vi "Lab Panel V5.23.vi"() -> ()   [LabVIEW 2013] (continued)
                    n2497 = local read "DISP LAB05-2"() -> (w4651:T4)
                    n2498 = local read "SIG LAB05-2"() -> (w4652:T2)
                    n2499 = local read "ON L05-2"() -> (w4648:cluster{"amps":dbl, "volts":dbl, "pf":dbl})
                    n2500 = Unbundle(w4652) -> ("AMPS"=w4658:dbl, "VOLTS"=w4656:dbl, "PF"=w4655:dbl, "Tmp Live"=w4654:dbl, "Tmp Neut"=w4657:dbl)
                    n2501 = Unbundle(w4651) -> ("CYCLE"=w4653:dbl)  [unwired: 2 out]
                    n2502 = stacked-sequence {
                      tunnel: w4658 -> [w4662 w4681]
                      tunnel: w4657 -> [_ w4680]
                      tunnel: w4656 -> [w4661 w4679]
                      tunnel: w4655 -> [w4660 w4678]
                      tunnel: w4654 -> [_ w4677]
                      tunnel: w4653 -> [_ w4676]
                      tunnel: w4650 -> [_ w4675]
                      tunnel: w4649 -> [w4663 _]
                      tunnel: w4648 -> [w4659 w4673]
                      tunnel: w4647 -> [_ w4674]
                      tunnel: w4646 -> [_ w4669]
                      frame #0 {
                        n2503 = case shown="True" w4663 {
                          tunnel: w4662 -> [_ w4668]
                          tunnel: w4661 -> [_ w4667]
                          tunnel: w4660 -> [_ w4666]
                          tunnel: w4659 -> [_ w4664]
                          frame False {
                          }
                          frame True {
                            n2504 = Bundle(cluster=w4664, "amps"=w4668, "volts"=w4667, "pf"=w4666) -> (w4665:cluster{"amps":dbl, "volts":dbl, "pf":dbl})
                            n2505 = local write "ON L05-2"(w4665) -> ()
                          }
                        }
                      }
                      frame #1 {
                        n2506 = Unbundle(w4673) -> ("amps"=w4672:dbl, "volts"=w4671:dbl, "pf"=w4670:dbl)
                        n2507 = case shown="True" w4674 {
                          tunnel: w4681 -> [_ w4713]
                          tunnel: w4680 -> [_ w4720]
                          tunnel: w4679 -> [_ _]
                          tunnel: w4678 -> [_ _]
                          tunnel: w4677 -> [_ w4719]
                          tunnel: w4676 -> [_ w4718]
                          tunnel: w4675 -> [_ w4683]
                          tunnel: w4672 -> [_ w4715]
                          tunnel: w4671 -> [_ w4714]
                          tunnel: w4670 -> [_ w4712]
                          tunnel: w4669 -> [_ w4704]
                          frame False {
                          }
                          frame True {
                            n2508 = local read "TDMS LAB05-2"() -> (w4717:refnum<k34>)
                            n2509 = Build Array(w4714) -> (w4709:dbl[])
                            n2510 = Build Array(w4712) -> (w4708:dbl[])
                            n2511 = Build Array(w4719) -> (w4707:dbl[])
                            n2512 = Build Array(w4720) -> (w4706:dbl[])
                            n2513 = Build Array(w4715) -> (w4711:dbl[])
                            n2514 = Build Array(w4713) -> (w4710:dbl[])
                            n2515 = Build Array(w4718) -> (w4705:dbl[])
                            n2516 = Build Array("AMPS ON", "AMPS OFF", "VOLTS", "PF", "TEMP Live", "TEMP Neut", "CYCLE") -> (w4688:string[])
                            n2517 = Bundle By Name("Y"=w4711, "t0"=w4704) -> (w4703:waveform(dbl))  [unwired: 1 in]
                            n2518 = Bundle By Name("Y"=w4710, "t0"=w4704) -> (w4702:waveform(dbl))  [unwired: 1 in]
                            n2519 = Bundle By Name("Y"=w4709, "t0"=w4704) -> (w4701:waveform(dbl))  [unwired: 1 in]
                            n2520 = Bundle By Name("Y"=w4708, "t0"=w4704) -> (w4700:waveform(dbl))  [unwired: 1 in]
                            n2521 = Bundle By Name("Y"=w4707, "t0"=w4704) -> (w4699:waveform(dbl))  [unwired: 1 in]
                            n2522 = Bundle By Name("Y"=w4706, "t0"=w4704) -> (w4698:waveform(dbl))  [unwired: 1 in]
                            n2523 = Bundle By Name("Y"=w4705, "t0"=w4704) -> (w4697:waveform(dbl))  [unwired: 1 in]
                            n2524 = Build Array(w4703, w4702, w4701, w4700, w4699, w4698, w4697) -> (w4696:waveform(dbl)[])
                            n2525 = TDMS Write(0:w4717, 5:"TEST VALUES", 7:w4688, 9:w4696) -> (4:w4687:refnum<k34>, 6:w4686:string, 15:w4685:errorcluster)  [unwired: 2 in, 1 out]
                            n2526 = TDMS Write(0:w4687, 5:w4686, 7:"TIME", 9:w4683, 11:w4685) -> (15:w4682:errorcluster)  [unwired: 1 in, 3 out]
                            n2527 = local write "data file error"(w4682) -> ()
                          }
                        }
                      }
                    }
                  }
                }
              }
            }
          }
          frame #13 {
            # "display test values on chart"
            n2528 = local read "jig cycle"() -> (w4725:dbl)
            n2529 = local read "on loops"() -> (w4727:dbl)
            n2530 = Add(x=w4727, y=2) -> (x+y=w4724:dbl)
            n2531 = Equal?(x=w4725, y=1) -> (x = y?=w4723:bool)
            n2532 = Equal?(x=w4725, y=w4724) -> (x = y?=w4722:bool)
            n2533 = Or(x=w4723, y=w4722) -> (x .or. y?=w4721:bool)
            "graph flag" <- w4721
            n2534 = global write "Global display 3.vi" "graph flag"(w4721) -> ()
            n2535 = case shown="True" w4721 {
              frame False {
              }
              frame True {
                n2536 = local read "SIG LAB05-1"() -> (w4770:T2)
                n2537 = local read "SIG LAB04-2"() -> (w4771:T2)
                n2538 = local read "SIG LAB05-2"() -> (w4769:T2)
                n2539 = local read "SIG LAB04-1"() -> (w4772:T2)
                n2540 = local read "SIG LAB03-1"() -> (w4774:T2)
                n2541 = local read "SIG LAB03-2"() -> (w4773:T2)
                n2542 = local read "SIG LAB01-1"() -> (w4778:T2)
                n2543 = local read "SIG LAB02-2"() -> (w4775:T2)
                n2544 = local read "SIG LAB02-1"() -> (w4776:T2)
                n2545 = local read "SIG LAB01-2"() -> (w4777:T2)
                n2546 = Unbundle(w4771) -> ("AMPS"=w4761:dbl, "VOLTS"=w4751:dbl, "Tmp Live"=w4741:dbl, "Tmp Neut"=w4731:dbl)  [unwired: 1 out]
                n2547 = Unbundle(w4770) -> ("AMPS"=w4760:dbl, "VOLTS"=w4750:dbl, "Tmp Live"=w4740:dbl, "Tmp Neut"=w4730:dbl)  [unwired: 1 out]
                n2548 = Unbundle(w4769) -> ("AMPS"=w4759:dbl, "VOLTS"=w4749:dbl, "Tmp Live"=w4739:dbl, "Tmp Neut"=w4729:dbl)  [unwired: 1 out]
                n2549 = Unbundle(w4772) -> ("AMPS"=w4762:dbl, "VOLTS"=w4752:dbl, "Tmp Live"=w4742:dbl, "Tmp Neut"=w4732:dbl)  [unwired: 1 out]
                n2550 = Unbundle(w4773) -> ("AMPS"=w4763:dbl, "VOLTS"=w4753:dbl, "Tmp Live"=w4743:dbl, "Tmp Neut"=w4733:dbl)  [unwired: 1 out]
                n2551 = Unbundle(w4774) -> ("AMPS"=w4764:dbl, "VOLTS"=w4754:dbl, "Tmp Live"=w4744:dbl, "Tmp Neut"=w4734:dbl)  [unwired: 1 out]
                n2552 = Unbundle(w4775) -> ("AMPS"=w4765:dbl, "VOLTS"=w4755:dbl, "Tmp Live"=w4745:dbl, "Tmp Neut"=w4735:dbl)  [unwired: 1 out]
                n2553 = Unbundle(w4776) -> ("AMPS"=w4766:dbl, "VOLTS"=w4756:dbl, "Tmp Live"=w4746:dbl, "Tmp Neut"=w4736:dbl)  [unwired: 1 out]
                n2554 = Unbundle(w4778) -> ("AMPS"=w4768:dbl, "VOLTS"=w4758:dbl, "Tmp Live"=w4748:dbl, "Tmp Neut"=w4738:dbl)  [unwired: 1 out]
                n2555 = Unbundle(w4777) -> ("AMPS"=w4767:dbl, "VOLTS"=w4757:dbl, "Tmp Live"=w4747:dbl, "Tmp Neut"=w4737:dbl)  [unwired: 1 out]
                n2556 = stacked-sequence {
                  tunnel: w4768 -> [w4810 _ _]
                  tunnel: w4767 -> [w4809 _ _]
                  tunnel: w4766 -> [w4800 _ _]
                  tunnel: w4765 -> [w4799 _ _]
                  tunnel: w4764 -> [w4789 _ _]
                  tunnel: w4763 -> [w4788 _ _]
                  tunnel: w4762 -> [_ w4833 _]
                  tunnel: w4761 -> [_ w4832 _]
                  tunnel: w4760 -> [_ w4822 _]
                  tunnel: w4759 -> [_ w4821 _]
                  tunnel: w4758 -> [w4807 _ _]
                  tunnel: w4757 -> [w4806 _ _]
                  tunnel: w4756 -> [w4797 _ _]
                  tunnel: w4755 -> [w4796 _ _]
                  tunnel: w4754 -> [w4787 _ _]
                  tunnel: w4753 -> [w4786 _ _]
                  tunnel: w4752 -> [_ w4831 _]
                  tunnel: w4751 -> [_ w4830 _]
                  tunnel: w4750 -> [_ w4820 _]
                  tunnel: w4749 -> [_ w4819 _]
                  tunnel: w4748 -> [w4804 _ _]
                  tunnel: w4747 -> [w4802 _ _]
                  tunnel: w4746 -> [w4793 _ _]
                  tunnel: w4745 -> [w4791 _ _]
                  tunnel: w4744 -> [w4785 _ _]
                  tunnel: w4743 -> [w4783 _ _]
                  tunnel: w4742 -> [_ w4829 _]
                  tunnel: w4741 -> [_ w4827 _]
                  tunnel: w4740 -> [_ w4818 _]
                  tunnel: w4739 -> [_ w4816 _]
                  tunnel: w4738 -> [w4803 _ _]
                  tunnel: w4737 -> [w4801 _ _]
                  tunnel: w4736 -> [w4792 _ _]
                  tunnel: w4735 -> [w4790 _ _]
                  tunnel: w4734 -> [w4784 _ _]
                  tunnel: w4733 -> [w4782 _ _]
                  tunnel: w4732 -> [_ w4828 _]
                  tunnel: w4731 -> [_ w4826 _]
                  tunnel: w4730 -> [_ w4817 _]
                  tunnel: w4729 -> [_ w4815 _]
                  frame #0 {
                    n2557 = Merge Signals(w4810, w4809) -> (→"LAB01 AMPS":dynamicdata)
                    n2558 = Merge Signals(w4807, w4806) -> (→"LAB01 VOLTS":dynamicdata)
                    n2559 = Merge Signals(w4787, w4786) -> (→"LAB03 VOLTS":dynamicdata)
                    n2560 = Merge Signals(w4804, w4803, w4802, w4801) -> (→"LAB01 deg C":dynamicdata)
                    n2561 = Merge Signals(w4800, w4799) -> (→"LAB02 AMPS":dynamicdata)
                    n2562 = Merge Signals(w4793, w4792, w4791, w4790) -> (→"LAB02 deg C":dynamicdata)
                    n2563 = Merge Signals(w4785, w4784, w4783, w4782) -> (→"LAB03 deg C":dynamicdata)
                    n2564 = Merge Signals(w4797, w4796) -> (→"LAB02 VOLTS":dynamicdata)
                    n2565 = Merge Signals(w4789, w4788) -> (→"LAB03 AMPS":dynamicdata)
                  }
                  frame #1 {
                    n2566 = Merge Signals(w4820, w4819) -> (→"LAB05 VOLTS":dynamicdata)
                    n2567 = Merge Signals(w4833, w4832) -> (→"LAB04 AMPS":dynamicdata)
                    n2568 = Merge Signals(w4822, w4821) -> (→"LAB05 AMPS":dynamicdata)
                    n2569 = Merge Signals(w4818, w4817, w4816, w4815) -> (→"LAB05 deg C":dynamicdata)
                    n2570 = Merge Signals(w4829, w4828, w4827, w4826) -> (→"LAB04 deg C":dynamicdata)
                    n2571 = Merge Signals(w4831, w4830) -> (→"LAB04 VOLTS":dynamicdata)
                  }
                  frame #2 {
                    n2572 = local read "LAB05 VOLTS"() -> (w4841:dynamicdata)
                    n2573 = local read "LAB04 VOLTS"() -> (w4842:dynamicdata)
                    n2574 = local read "LAB02 VOLTS"() -> (w4844:dynamicdata)
                    n2575 = local read "LAB03 VOLTS"() -> (w4843:dynamicdata)
                    n2576 = local read "LAB05 AMPS"() -> (w4847:dynamicdata)
                    n2577 = local read "LAB01 VOLTS"() -> (w4845:dynamicdata)
                    n2578 = local read "LAB04 AMPS"() -> (w4848:dynamicdata)
                    n2579 = local read "LAB03 AMPS"() -> (w4849:dynamicdata)
                    n2580 = local read "LAB03 deg C"() -> (w4837:dynamicdata)
                    n2581 = local read "LAB02 AMPS"() -> (w4850:dynamicdata)
                    n2582 = local read "LAB04 deg C"() -> (w4836:dynamicdata)
                    n2583 = local read "LAB05 deg C"() -> (w4835:dynamicdata)
                    n2584 = local read "LAB02 deg C"() -> (w4838:dynamicdata)
                    n2585 = local read "LAB01 deg C"() -> (w4839:dynamicdata)
                    n2586 = local read "LAB01 AMPS"() -> (w4851:dynamicdata)
                    n2587 = Merge Signals(w4839, w4838, w4837, w4836, w4835) -> (w4834:dynamicdata)
                    n2588 = Merge Signals(w4851, w4850, w4849, w4848, w4847) -> (w4846:dynamicdata)
                    n2589 = Merge Signals(w4845, w4844, w4843, w4842, w4841) -> (w4840:dynamicdata)
                    n2590 = global write "Global display 3.vi" "graph volts"(w4840) -> ()
                    n2591 = global write "Global display 3.vi" "graph deg C"(w4834) -> ()
                    n2592 = global write "Global display 3.vi" "graph amps"(w4846) -> ()
                  }
                }
              }
            }
          }
          frame #14 {
            # "check for amps fail"
            # "check for cycle test & temperature rise fail conditions"
            n2593 = local read "on loops"() -> (w4878:dbl)
            n2594 = local read "jig cycle"() -> (w4875:dbl)
            n2595 = local read "jig cycle"() -> (w4880:dbl)
            n2596 = Add(x=w4878, y=3.0) -> (x+y=w4876:dbl)
            n2597 = Equal?(x=w4875, y=w4876) -> (x = y?=w4871:bool)
            n2598 = local read "Fail Loops"() -> (w4852:dbl)
            n2599 = Equal?(x=w4880, y=1.0) -> (x = y?=w4873:bool)
            n2600 = global write "Global 1.vi" "fail count"(w4852) -> ()
            n2601 = stacked-sequence {
              tunnel: w4874 -> [w4883 _ _ _ _ _ _ _ _ _]
              tunnel: w4873 -> [w4884 w4904 w4924 w4944 w4964 w4984 w5004 w5024 w5044 w5064]
              tunnel: w4872 -> [w4881 _ _ _ _ _ _ _ _ _]
              tunnel: w4871 -> [w4882 w4903 w4923 w4943 w4963 w4983 w5003 w5023 w5043 w5063]
              tunnel: w4870 -> [_ w4902 _ _ _ _ _ _ _ _]
              tunnel: w4869 -> [_ w4901 _ _ _ _ _ _ _ _]
              tunnel: w4868 -> [_ _ w4922 _ _ _ _ _ _ _]
              tunnel: w4867 -> [_ _ w4921 _ _ _ _ _ _ _]
              tunnel: w4866 -> [_ _ _ w4942 _ _ _ _ _ _]
              tunnel: w4865 -> [_ _ _ w4941 _ _ _ _ _ _]
              tunnel: w4864 -> [_ _ _ _ w4962 _ _ _ _ _]
              tunnel: w4863 -> [_ _ _ _ w4961 _ _ _ _ _]
              tunnel: w4862 -> [_ _ _ _ _ w4982 _ _ _ _]
              tunnel: w4861 -> [_ _ _ _ _ w4981 _ _ _ _]
              tunnel: w4860 -> [_ _ _ _ _ _ w5002 _ _ _]
              tunnel: w4859 -> [_ _ _ _ _ _ w5001 _ _ _]
              tunnel: w4858 -> [_ _ _ _ _ _ _ w5022 _ _]
              tunnel: w4857 -> [_ _ _ _ _ _ _ w5021 _ _]
              tunnel: w4856 -> [_ _ _ _ _ _ _ _ w5042 _]
              tunnel: w4855 -> [_ _ _ _ _ _ _ _ w5041 _]
              tunnel: w4854 -> [_ _ _ _ _ _ _ _ _ w5062]
              tunnel: w4853 -> [_ _ _ _ _ _ _ _ _ w5061]
              frame #0 {
                # "LAB01-1"
                n2602 = case shown="True" w4881 {
                  tunnel: w4884 -> [_ w4897]
                  tunnel: w4883 -> [_ w4894]
                  tunnel: w4882 -> [_ w4893]
                  frame False {
                  }
                  frame True {
                    n2603 = local read "TEMP START LAB01-1"() -> (w4899:cluster{"TL":dbl, "TN":dbl})
                    n2604 = local read "RESULT LAB01-1"() -> (w4888:bool)
                    n2605 = local read "FAIL LAB01-1"() -> (w4891:cluster{"LO":dbl, "HI":dbl})
                    n2606 = local read "TDMS LAB01-1"() -> (w4898:refnum<k34>)
                    n2607 = local read "SET LAB01-1"() -> (w4895:T5)
                    n2608 = local read "DISP LAB01-1"() -> (w4896:T4)
                    n2609 = local read "SIG LAB01-1"() -> (w4900:T2)
                    n2610 = Bundle("FAIL LAB01-1"=w4891, "SIG LAB01-1"=w4900, "TEMP START LAB01-1"=w4899, "DISP LAB01-1"=w4896, "SET LAB01-1"=w4895, "TDMS LAB01-1"=w4898) -> (w4885:T33)  [unwired: 1 in]
                    n2611 = call "sub vi - cycle&temp fail v7.vi"("Amps Lo?"=w4897, "Input Cluster"=w4885, "SELECT"=w4894, "Amps Hi?"=w4893, "Result In"=w4888) -> ("(FAIL) out"=w4890:cluster{"FAIL LO":dbl, "FAIL HI":dbl}, "(DISP) out"=w4886:T4, "T-RISE"=w4887:cluster{"T-RISE (L)":dbl, "T-RISE (N)":dbl}, "Result Out"=w4889:bool, "file error"=w4892:errorcluster)  [unwired: 10 in]
                    n2612 = local write "TEMP RISE LAB01-1"(w4887) -> ()
                    n2613 = local write "FAIL LAB01-1"(w4890) -> ()
                    n2614 = local write "DISP LAB01-1"(w4886) -> ()
                    n2615 = local write "RESULT LAB01-1"(w4889) -> ()
                    n2616 = local write "data file error"(w4892) -> ()
                  }
                }
              }
              frame #1 {
                # "LAB01-2"
                n2617 = case shown="True" w4902 {
                  tunnel: w4904 -> [_ w4917]
                  tunnel: w4901 -> [_ w4914]
                  tunnel: w4903 -> [_ w4913]
                  frame False {
                  }
                  frame True {
                    n2618 = local read "TEMP START LAB01-2"() -> (w4919:cluster{"TL":dbl, "TN":dbl})
                    n2619 = local read "FAIL LAB01-2"() -> (w4910:cluster{"LO":dbl, "HI":dbl})
                    n2620 = local read "TDMS LAB01-2"() -> (w4918:refnum<k34>)
                    n2621 = local read "SET LAB01-2"() -> (w4915:T5)
                    n2622 = local read "DISP LAB01-2"() -> (w4916:T4)
                    n2623 = local read "RESULT LAB01-2"() -> (w4907:bool)
                    n2624 = local read "SIG LAB01-2"() -> (w4920:T2)
                    n2625 = Bundle("FAIL LAB01-2"=w4910, "SIG LAB01-2"=w4920, "TEMP START LAB01-2"=w4919, "DISP LAB01-2"=w4916, "SET LAB01-2"=w4915, "TDMS LAB01-2"=w4918) -> (w4905:T34)  [unwired: 1 in]
                    n2626 = call "sub vi - cycle&temp fail v7.vi"("Amps Lo?"=w4917, "Input Cluster"=w4905, "SELECT"=w4914, "Amps Hi?"=w4913, "Result In"=w4907) -> ("(FAIL) out"=w4909:cluster{"FAIL LO":dbl, "FAIL HI":dbl}, "(DISP) out"=w4912:T4, "T-RISE"=w4906:cluster{"T-RISE (L)":dbl, "T-RISE (N)":dbl}, "Result Out"=w4908:bool, "file error"=w4911:errorcluster)  [unwired: 10 in]
                    n2627 = local write "TEMP RISE LAB01-2"(w4906) -> ()
                    n2628 = local write "FAIL LAB01-2"(w4909) -> ()
                    n2629 = local write "DISP LAB01-2"(w4912) -> ()
                    n2630 = local write "RESULT LAB01-2"(w4908) -> ()
                    n2631 = local write "data file error"(w4911) -> ()
                  }
                }
              }
              frame #2 {
                # "LAB02-1"
                n2632 = case shown="True" w4922 {
                  tunnel: w4924 -> [_ w4937]
                  tunnel: w4921 -> [_ w4934]
                  tunnel: w4923 -> [_ w4933]
                  frame False {
                  }
                  frame True {
                    n2633 = local read "TEMP START LAB02-1"() -> (w4939:cluster{"TL":dbl, "TN":dbl})
                    n2634 = local read "FAIL LAB02-1"() -> (w4930:cluster{"LO":dbl, "HI":dbl})
                    n2635 = local read "TDMS LAB02-1"() -> (w4938:refnum<k34>)
                    n2636 = local read "SET LAB02-1"() -> (w4935:T5)
                    n2637 = local read "DISP LAB02-1"() -> (w4936:T4)
                    n2638 = local read "SIG LAB02-1"() -> (w4940:T2)
                    n2639 = local read "RESULT LAB02-1"() -> (w4927:bool)
                    n2640 = Bundle("FAIL LAB02-1"=w4930, "SIG LAB02-1"=w4940, "TEMP START LAB02-1"=w4939, "DISP LAB02-1"=w4936, "SET LAB02-1"=w4935, "TDMS LAB02-1"=w4938) -> (w4925:T35)  [unwired: 1 in]
                    n2641 = call "sub vi - cycle&temp fail v7.vi"("Amps Lo?"=w4937, "Input Cluster"=w4925, "SELECT"=w4934, "Amps Hi?"=w4933, "Result In"=w4927) -> ("(FAIL) out"=w4929:cluster{"FAIL LO":dbl, "FAIL HI":dbl}, "(DISP) out"=w4932:T4, "T-RISE"=w4926:cluster{"T-RISE (L)":dbl, "T-RISE (N)":dbl}, "Result Out"=w4928:bool, "file error"=w4931:errorcluster)  [unwired: 10 in]
                    n2642 = local write "TEMP RISE LAB02-1"(w4926) -> ()
                    n2643 = local write "FAIL LAB02-1"(w4929) -> ()
                    n2644 = local write "DISP LAB02-1"(w4932) -> ()
                    n2645 = local write "RESULT LAB02-1"(w4928) -> ()
                    n2646 = local write "data file error"(w4931) -> ()
                  }
                }
              }
              frame #3 {
                # "LAB02-2"
                n2647 = case shown="True" w4942 {
                  tunnel: w4944 -> [_ w4957]
                  tunnel: w4941 -> [_ w4954]
                  tunnel: w4943 -> [_ w4953]
                  frame False {
                  }
                  frame True {
                    n2648 = local read "TEMP START LAB02-2"() -> (w4959:cluster{"TL":dbl, "TN":dbl})
                    n2649 = local read "FAIL LAB02-2"() -> (w4950:cluster{"LO":dbl, "HI":dbl})
                    n2650 = local read "TDMS LAB02-2"() -> (w4958:refnum<k34>)
                    n2651 = local read "SET LAB02-2"() -> (w4955:T5)
                    n2652 = local read "DISP LAB02-2"() -> (w4956:T4)
                    n2653 = local read "SIG LAB02-2"() -> (w4960:T2)
                    n2654 = local read "RESULT LAB02-2"() -> (w4947:bool)
                    n2655 = Bundle("FAIL LAB02-2"=w4950, "SIG LAB02-2"=w4960, "TEMP START LAB02-2"=w4959, "DISP LAB02-2"=w4956, "SET LAB02-2"=w4955, "TDMS LAB02-2"=w4958) -> (w4945:T36)  [unwired: 1 in]
                    n2656 = call "sub vi - cycle&temp fail v7.vi"("Amps Lo?"=w4957, "Input Cluster"=w4945, "SELECT"=w4954, "Amps Hi?"=w4953, "Result In"=w4947) -> ("(FAIL) out"=w4949:cluster{"FAIL LO":dbl, "FAIL HI":dbl}, "(DISP) out"=w4952:T4, "T-RISE"=w4946:cluster{"T-RISE (L)":dbl, "T-RISE (N)":dbl}, "Result Out"=w4948:bool, "file error"=w4951:errorcluster)  [unwired: 10 in]
                    n2657 = local write "TEMP RISE LAB02-2"(w4946) -> ()
                    n2658 = local write "FAIL LAB02-2"(w4949) -> ()
                    n2659 = local write "DISP LAB02-2"(w4952) -> ()
                    n2660 = local write "RESULT LAB02-2"(w4948) -> ()
                    n2661 = local write "data file error"(w4951) -> ()
                  }
                }
              }
              frame #4 {
                # "LAB03-1"
                n2662 = case shown="True" w4962 {
                  tunnel: w4964 -> [_ w4977]
                  tunnel: w4961 -> [_ w4974]
                  tunnel: w4963 -> [_ w4973]
                  frame False {
                  }
                  frame True {
                    n2663 = local read "TEMP START LAB03-1"() -> (w4979:cluster{"TL":dbl, "TN":dbl})
                    n2664 = local read "FAIL LAB03-1"() -> (w4970:cluster{"LO":dbl, "HI":dbl})
                    n2665 = local read "TDMS LAB03-1"() -> (w4978:refnum<k34>)
                    n2666 = local read "SET LAB03-1"() -> (w4975:T5)
                    n2667 = local read "DISP LAB03-1"() -> (w4976:T4)
                    n2668 = local read "SIG LAB03-1"() -> (w4980:T2)
                    n2669 = local read "RESULT LAB03-1"() -> (w4967:bool)
                    n2670 = Bundle("FAIL LAB03-1"=w4970, "SIG LAB03-1"=w4980, "TEMP START LAB03-1"=w4979, "DISP LAB03-1"=w4976, "SET LAB03-1"=w4975, "TDMS LAB03-1"=w4978) -> (w4965:T37)  [unwired: 1 in]
                    n2671 = call "sub vi - cycle&temp fail v7.vi"("Amps Lo?"=w4977, "Input Cluster"=w4965, "SELECT"=w4974, "Amps Hi?"=w4973, "Result In"=w4967) -> ("(FAIL) out"=w4969:cluster{"FAIL LO":dbl, "FAIL HI":dbl}, "(DISP) out"=w4972:T4, "T-RISE"=w4966:cluster{"T-RISE (L)":dbl, "T-RISE (N)":dbl}, "Result Out"=w4968:bool, "file error"=w4971:errorcluster)  [unwired: 10 in]
                    n2672 = local write "TEMP RISE LAB03-1"(w4966) -> ()
                    n2673 = local write "FAIL LAB03-1"(w4969) -> ()
                    n2674 = local write "DISP LAB03-1"(w4972) -> ()
                    n2675 = local write "RESULT LAB03-1"(w4968) -> ()
                    n2676 = local write "data file error"(w4971) -> ()
                  }
                }
              }
              frame #5 {
                # "LAB03-2"
                n2677 = case shown="True" w4982 {
                  tunnel: w4984 -> [_ w4997]
                  tunnel: w4981 -> [_ w4994]
                  tunnel: w4983 -> [_ w4993]
                  frame False {
                  }
                  frame True {
                    n2678 = local read "TEMP START LAB03-2"() -> (w4999:cluster{"TL":dbl, "TN":dbl})
                    n2679 = local read "FAIL LAB03-2"() -> (w4990:cluster{"LO":dbl, "HI":dbl})
                    n2680 = local read "TDMS LAB03-2"() -> (w4998:refnum<k34>)
                    n2681 = local read "SET LAB03-2"() -> (w4995:T5)
                    n2682 = local read "DISP LAB03-2"() -> (w4996:T4)
                    n2683 = local read "RESULT LAB03-2"() -> (w4987:bool)
                    n2684 = local read "SIG LAB03-2"() -> (w5000:T2)
                    n2685 = Bundle("FAIL LAB03-2"=w4990, "SIG LAB03-2"=w5000, "TEMP START LAB03-2"=w4999, "DISP LAB03-2"=w4996, "SET LAB03-2"=w4995, "TDMS LAB03-2"=w4998) -> (w4985:T38)  [unwired: 1 in]
                    n2686 = call "sub vi - cycle&temp fail v7.vi"("Amps Lo?"=w4997, "Input Cluster"=w4985, "SELECT"=w4994, "Amps Hi?"=w4993, "Result In"=w4987) -> ("(FAIL) out"=w4989:cluster{"FAIL LO":dbl, "FAIL HI":dbl}, "(DISP) out"=w4992:T4, "T-RISE"=w4986:cluster{"T-RISE (L)":dbl, "T-RISE (N)":dbl}, "Result Out"=w4988:bool, "file error"=w4991:errorcluster)  [unwired: 10 in]
                    n2687 = local write "FAIL LAB03-2"(w4989) -> ()
                    n2688 = local write "TEMP RISE LAB03-2"(w4986) -> ()
                    n2689 = local write "DISP LAB03-2"(w4992) -> ()
                    n2690 = local write "RESULT LAB03-2"(w4988) -> ()
                    n2691 = local write "data file error"(w4991) -> ()
                  }
                }
              }
              frame #6 {
                # "LAB04-1"
                n2692 = case shown="True" w5002 {
                  tunnel: w5004 -> [_ w5017]
                  tunnel: w5001 -> [_ w5014]
                  tunnel: w5003 -> [_ w5013]
                  frame False {
                  }
                  frame True {
                    n2693 = local read "TEMP START LAB04-1"() -> (w5019:cluster{"TL":dbl, "TN":dbl})
                    n2694 = local read "FAIL LAB04-1"() -> (w5010:cluster{"LO":dbl, "HI":dbl})
                    n2695 = local read "TDMS LAB04-1"() -> (w5018:refnum<k34>)
                    n2696 = local read "SET LAB04-1"() -> (w5015:T5)
                    n2697 = local read "DISP LAB04-1"() -> (w5016:T4)
                    n2698 = local read "SIG LAB04-1"() -> (w5020:T2)
                    n2699 = local read "RESULT LAB04-1"() -> (w5007:bool)
                    n2700 = Bundle("FAIL LAB04-1"=w5010, "SIG LAB04-1"=w5020, "TEMP START LAB04-1"=w5019, "DISP LAB04-1"=w5016, "SET LAB04-1"=w5015, "TDMS LAB04-1"=w5018) -> (w5005:T39)  [unwired: 1 in]
                    n2701 = call "sub vi - cycle&temp fail v7.vi"("Amps Lo?"=w5017, "Input Cluster"=w5005, "SELECT"=w5014, "Amps Hi?"=w5013, "Result In"=w5007) -> ("(FAIL) out"=w5009:cluster{"FAIL LO":dbl, "FAIL HI":dbl}, "(DISP) out"=w5012:T4, "T-RISE"=w5006:cluster{"T-RISE (L)":dbl, "T-RISE (N)":dbl}, "Result Out"=w5008:bool, "file error"=w5011:errorcluster)  [unwired: 10 in]
                    n2702 = local write "TEMP RISE LAB04-1"(w5006) -> ()
                    n2703 = local write "FAIL LAB04-1"(w5009) -> ()
                    n2704 = local write "DISP LAB04-1"(w5012) -> ()
                    n2705 = local write "RESULT LAB04-1"(w5008) -> ()
                    n2706 = local write "data file error"(w5011) -> ()
                  }
                }
              }
              frame #7 {
                # "LAB04-2"
                n2707 = case shown="True" w5022 {
                  tunnel: w5024 -> [_ w5037]
                  tunnel: w5021 -> [_ w5034]
                  tunnel: w5023 -> [_ w5033]
                  frame False {
                  }
                  frame True {
                    n2708 = local read "TEMP START LAB04-2"() -> (w5039:cluster{"TL":dbl, "TN":dbl})
                    n2709 = local read "FAIL LAB04-2"() -> (w5030:cluster{"LO":dbl, "HI":dbl})
                    n2710 = local read "TDMS LAB04-2"() -> (w5038:refnum<k34>)
                    n2711 = local read "SET LAB04-2"() -> (w5035:T5)
                    n2712 = local read "DISP LAB04-2"() -> (w5036:T4)
                    n2713 = local read "SIG LAB04-2"() -> (w5040:T2)
                    n2714 = local read "RESULT LAB04-2"() -> (w5027:bool)
                    n2715 = Bundle("FAIL LAB04-2"=w5030, "SIG LAB04-2"=w5040, "TEMP START LAB04-2"=w5039, "DISP LAB04-2"=w5036, "SET LAB04-2"=w5035, "TDMS LAB04-2"=w5038) -> (w5025:T40)  [unwired: 1 in]
                    n2716 = call "sub vi - cycle&temp fail v7.vi"("Amps Lo?"=w5037, "Input Cluster"=w5025, "SELECT"=w5034, "Amps Hi?"=w5033, "Result In"=w5027) -> ("(FAIL) out"=w5029:cluster{"FAIL LO":dbl, "FAIL HI":dbl}, "(DISP) out"=w5032:T4, "T-RISE"=w5026:cluster{"T-RISE (L)":dbl, "T-RISE (N)":dbl}, "Result Out"=w5028:bool, "file error"=w5031:errorcluster)  [unwired: 10 in]
                    n2717 = local write "TEMP RISE LAB04-2"(w5026) -> ()
                    n2718 = local write "FAIL LAB04-2"(w5029) -> ()
                    n2719 = local write "DISP LAB04-2"(w5032) -> ()
                    n2720 = local write "RESULT LAB04-2"(w5028) -> ()
                    n2721 = local write "data file error"(w5031) -> ()
                  }
                }
              }
              frame #8 {
                # "LAB05-1"
                n2722 = case shown="True" w5042 {
                  tunnel: w5044 -> [_ w5057]
                  tunnel: w5041 -> [_ w5054]
                  tunnel: w5043 -> [_ w5053]
                  frame False {
                  }
                  frame True {
                    n2723 = local read "TEMP START LAB05-1"() -> (w5059:cluster{"TL":dbl, "TN":dbl})
                    n2724 = local read "FAIL LAB05-1"() -> (w5050:cluster{"LO":dbl, "HI":dbl})
                    n2725 = local read "TDMS LAB05-1"() -> (w5058:refnum<k34>)
                    n2726 = local read "SET LAB05-1"() -> (w5055:T5)
                    n2727 = local read "DISP LAB05-1"() -> (w5056:T4)
                    n2728 = local read "SIG LAB05-1"() -> (w5060:T2)
                    n2729 = local read "RESULT LAB05-1"() -> (w5047:bool)
                    n2730 = Bundle("FAIL LAB05-1"=w5050, "SIG LAB05-1"=w5060, "TEMP START LAB05-1"=w5059, "DISP LAB05-1"=w5056, "SET LAB05-1"=w5055, "TDMS LAB05-1"=w5058) -> (w5045:T41)  [unwired: 1 in]
                    n2731 = call "sub vi - cycle&temp fail v7.vi"("Amps Lo?"=w5057, "Input Cluster"=w5045, "SELECT"=w5054, "Amps Hi?"=w5053, "Result In"=w5047) -> ("(FAIL) out"=w5049:cluster{"FAIL LO":dbl, "FAIL HI":dbl}, "(DISP) out"=w5052:T4, "T-RISE"=w5046:cluster{"T-RISE (L)":dbl, "T-RISE (N)":dbl}, "Result Out"=w5048:bool, "file error"=w5051:errorcluster)  [unwired: 10 in]
                    n2732 = local write "TEMP RISE LAB05-1"(w5046) -> ()
                    n2733 = local write "FAIL LAB05-1"(w5049) -> ()
                    n2734 = local write "DISP LAB05-1"(w5052) -> ()
                    n2735 = local write "RESULT LAB05-1"(w5048) -> ()
                    n2736 = local write "data file error"(w5051) -> ()
                  }
                }
              }
              frame #9 {
                # "LAB05-2"
                n2737 = case shown="True" w5062 {
                  tunnel: w5064 -> [_ w5077]
                  tunnel: w5061 -> [_ w5074]
                  tunnel: w5063 -> [_ w5073]
                  frame False {
                  }
                  frame True {
                    n2738 = local read "TEMP START LAB05-2"() -> (w5079:cluster{"TL":dbl, "TN":dbl})
                    n2739 = local read "FAIL LAB05-2"() -> (w5070:cluster{"LO":dbl, "HI":dbl})
                    n2740 = local read "TDMS LAB05-2"() -> (w5078:refnum<k34>)
                    n2741 = local read "SET LAB05-2"() -> (w5075:T5)
                    n2742 = local read "DISP LAB05-2"() -> (w5076:T4)
                    n2743 = local read "SIG LAB05-2"() -> (w5080:T2)
                    n2744 = local read "RESULT LAB05-2"() -> (w5067:bool)
                    n2745 = Bundle("FAIL LAB05-2"=w5070, "SIG LAB05-2"=w5080, "TEMP START LAB05-2"=w5079, "DISP LAB05-2"=w5076, "SET LAB05-2"=w5075, "TDMS LAB05-2"=w5078) -> (w5065:T42)  [unwired: 1 in]
                    n2746 = call "sub vi - cycle&temp fail v7.vi"("Amps Lo?"=w5077, "Input Cluster"=w5065, "SELECT"=w5074, "Amps Hi?"=w5073, "Result In"=w5067) -> ("(FAIL) out"=w5069:cluster{"FAIL LO":dbl, "FAIL HI":dbl}, "(DISP) out"=w5072:T4, "T-RISE"=w5066:cluster{"T-RISE (L)":dbl, "T-RISE (N)":dbl}, "Result Out"=w5068:bool, "file error"=w5071:errorcluster)  [unwired: 10 in]
                    n2747 = local write "TEMP RISE LAB05-2"(w5066) -> ()
                    n2748 = local write "FAIL LAB05-2"(w5069) -> ()
                    n2749 = local write "DISP LAB05-2"(w5072) -> ()
                    n2750 = local write "RESULT LAB05-2"(w5068) -> ()
                    n2751 = local write "data file error"(w5071) -> ()
                  }
                }
              }
            }
          }
          frame #15 {
            # "run calibration routine"
            n2752 = local read "SET (cal)"() -> (w5081:bool)
            n2753 = case shown="True" w5081 {
              frame False {
              }
              frame True {
                n2754 = stacked-sequence {
                  seq-local: [w5082 _ _] -> [_ w5084 _]
                  frame #0 {
                    n2755 = call "CALIBRATION PASSWORD"() -> ("PASSWORD"=w5082:string)  [unwired: 17 in, 2 out]
                  }
                  frame #1 {
                    n2756 = Equal?(x=w5084, y="7777") -> (x = y?=w5083:bool)
                    n2757 = case shown="True" w5083 {
                      frame False {
                      }
                      frame True {
                        n2758 = stacked-sequence {
                          frame #0 {
                            n2759 = local read "Temp Test Cal"() -> (w5086:dbl)
                            n2760 = call "sub vi - calibration v1.vi"("Temp Test Cal"=w5086) -> ()  [unwired: 11 in]
                          }
                          frame #1 {
                            n2761 = call "sub vi - get calibration values v1.vi"() -> ("TEMP REF CAL"=w5087:dbl, "LAB01 (CAL)"=w5092:T14, "LAB02 (CAL)"=w5091:T15, "LAB03 (CAL)"=w5090:T14, "LAB04 (CAL)"=w5089:T14, "calibration file error out"=w5093:errorcluster, "LAB05 (CAL)"=w5088:T14)  [unwired: 9 in]
                            n2762 = local write "TEMP REF cal"(w5087) -> ()
                            n2763 = local write "cal file error out"(w5093) -> ()
                            n2764 = local write "CAL LAB04"(w5089) -> ()
                            n2765 = local write "CAL LAB05"(w5088) -> ()
                            n2766 = local write "CAL LAB01"(w5092) -> ()
                            n2767 = local write "CAL LAB02"(w5091) -> ()
                            n2768 = local write "CAL LAB03"(w5090) -> ()
                          }
                        }
                      }
                    }
                  }
                  frame #2 {
                    n2769 = local write "SET (cal)"(FALSE) -> ()
                  }
                }
              }
            }
          }
          frame #16 {
            # "save certain settings to file"
            n2770 = String To Path(string="c:\\crabtree\\Set Up\\") -> (path=w5096:path)
            n2771 = Build Path(base path=w5096, name or relative path="settings.bin") -> (appended path=w5098:path)
            n2772 = Build Path(base path=w5096, name or relative path="mail.bin") -> (appended path=w5095:path)
            n2773 = Create Folder(path (use dialog)=w5096) -> (error out=w5101:errorcluster)  [unwired: 2 in, 2 out]
            n2774 = call <vilib>:"Clear Errors.vi"("error in (no error)"=w5101) -> ()  [unwired: 6 in, 1 out]
            n2775 = stacked-sequence {
              seq-local: [w5113 _] -> [_ w5126]
              tunnel: w5098 -> [_ w5127]
              tunnel: w5095 -> [_ w5125]
              frame #0 {
                n2776 = local read "C drive data root dir"() -> (w5112:path)
                n2777 = local read "Select COM port"() -> (w5109:refnum<visa-resource-name>)
                n2778 = local read "Network Directory"() -> (w5118:path)
                n2779 = local read "SET LAB05-2"() -> (w5117:T5)
                n2780 = local read "SET LAB05-1"() -> (w5116:T5)
                n2781 = local read "SET LAB04-2"() -> (w5115:T5)
                n2782 = local read "SET LAB03-2"() -> (w5119:T5)
                n2783 = local read "SET LAB04-1"() -> (w5114:T5)
                n2784 = local read "SET LAB03-1"() -> (w5120:T5)
                n2785 = local read "SET LAB02-2"() -> (w5121:T5)
                n2786 = local read "SET LAB02-1"() -> (w5122:T5)
                n2787 = local read "Temp Delay Lps"() -> (w5108:dbl)
                n2788 = local read "Amps Fail level"() -> (w5104:dbl)
                n2789 = local read "SET LAB01-2"() -> (w5123:T5)
                n2790 = local read "Temp Test Cal"() -> (w5105:dbl)
                n2791 = local read "SET LAB01-1"() -> (w5124:T5)
                n2792 = local read "Mail Test File To:"() -> (w5103:string)
                n2793 = local read "Temp Value"() -> (w5107:dbl)
                n2794 = local read "Fail Loops"() -> (w5106:dbl)
                n2795 = local read "Mail Test Fail"() -> (w5102:bool)
                n2796 = local read "RATE (Hz)"() -> (w5111:dbl)
                n2797 = local read "SAMPLES"() -> (w5110:dbl)
                n2798 = Bundle("SET LAB01-1"=w5124, "SET LAB01-2"=w5123, "SET LAB02-1"=w5122, "SET LAB02-2"=w5121, "SET LAB03-1"=w5120, "SET LAB03-2"=w5119, "SET LAB04-1"=w5114, "SET LAB04-2"=w5115, "SET LAB05-1"=w5116, "SET LAB05-2"=w5117, "Network Directory"=w5118, "C drive data root dir"=w5112, "RATE (Hz)"=w5111, "SAMPLES"=w5110, "Select COM port"=w5109, "Temp Delay Lps"=w5108, "Temp Value"=w5107, "Fail Loops"=w5106, "Temp Test Cal"=w5105, "Amps Fail level"=w5104, "Mail Test File To:"=w5103, "Mail Test Fail"=w5102) -> (w5113:T22)  [unwired: 1 in]
              }
              frame #1 {
                n2799 = event shown="[1] \"SET LAB01-1\", \"SET LAB01-2\", \"SET LAB02-1\", \"SET LAB02-2\", \"SET LAB03-1\", \"SET LAB03-2\", \"SET LAB04-1\", \"SET LAB04-2\", \"SET LAB05-1\", \"SET LAB05-2\", \"Network Directory\", \"C drive data root dir\", \"RATE (Hz)\", \"SAMPLES\", \"Select COM port\", \"Temp Delay Lps\", \"Temp Value\", \"Fail Loops\", \"Temp Test Cal\", \"Amps Fail level\", \"Mail Test File To:\", \"Mail Test Fail\": Value Change" {
                  selector: _ -> [_ _ _]
                  dyn-events: _ -> [_ _ _]
                  timeout: 10.0 -> [_ _ _]
                  tunnel: w5127 -> [_ w5129 _]
                  tunnel: w5126 -> [_ w5130 _]
                  tunnel: w5125 -> [_ _ w5141]
                  event Timeout {
                    n2800 = event-data() -> ()  [unwired: 1 in, 3 out]
                  }
                  event "SET LAB01-1", "SET LAB01-2", "SET LAB02-1", "SET LAB02-2", "SET LAB03-1", "SET LAB03-2", "SET LAB04-1", "SET LAB04-2", "SET LAB05-1", "SET LAB05-2", "Network Directory", "C drive data root dir", "RATE (Hz)", "SAMPLES", "Select COM port", "Temp Delay Lps", "Temp Value", "Fail Loops", "Temp Test Cal", "Amps Fail level", "Mail Test File To:", "Mail Test Fail": Value Change {
                    n2801 = event-data() -> ()  [unwired: 1 in, 6 out]
                    n2802 = Open/Create/Replace File(file path (use dialog)=w5129, operation (0:open)=T17."replace or create") -> (refnum out=w5135:refnum<file>, error out=w5134:errorcluster)  [unwired: 4 in, 1 out]
                    n2803 = Write to Binary File(file (use dialog)=w5135, data=w5130, error in=w5134) -> (refnum out=w5133:refnum<file>, error out=w5132:errorcluster)  [unwired: 3 in, 1 out]
                    n2804 = Close File(refnum=w5133, error in=w5132) -> (error out=w5131:errorcluster)  [unwired: 1 out]
                    n2805 = local write "data file error"(w5131) -> ()
                  }
                  event "MAIL SETTINGS.OUT SERVER ADDRESS", "MAIL SETTINGS.FROM ACCOUNT", "MAIL SETTINGS.USER NAME", "MAIL SETTINGS.PASSWORD", "Auto Mail Send", "TO (string):": Value Change {
                    n2806 = event-data() -> ()  [unwired: 1 in, 6 out]
                    n2807 = local read "MAIL SETTINGS"() -> (w5140:T7)
                    n2808 = local read "Auto Mail Send"() -> (w5138:bool)
                    n2809 = local read "TO (string):"() -> (w5137:string)
                    n2810 = Open/Create/Replace File(file path (use dialog)=w5141, operation (0:open)=T17."replace or create") -> (refnum out=w5146:refnum<file>, error out=w5145:errorcluster)  [unwired: 4 in, 1 out]
                    n2811 = Bundle("MAIL SETTINGS"=w5140, "Auto Mail Send"=w5138, "TO (string):"=w5137) -> (w5139:T43)  [unwired: 1 in]
                    n2812 = Write to Binary File(file (use dialog)=w5146, data=w5139, error in=w5145) -> (refnum out=w5144:refnum<file>, error out=w5143:errorcluster)  [unwired: 3 in, 1 out]
                    n2813 = Close File(refnum=w5144, error in=w5143) -> (error out=w5142:errorcluster)  [unwired: 1 out]
                    n2814 = local write "data file error"(w5142) -> ()
                  }
                }
              }
            }
          }
          frame #17 {
            # "mail control"
            n2815 = local read "MAIL SETTINGS"() -> (w5163:T7)
            n2816 = local read "Auto Mail Send"() -> (w5149:bool)
            n2817 = Unbundle(w5163) -> ("OUT SERVER ADDRESS"=w5162:string, "FROM ACCOUNT"=w5161:string, "TEST MAIL"=w5160:bool)  [unwired: 4 out]
            n2818 = stacked-sequence {
              tunnel: "TO (string):" -> [_ w5202]
              tunnel: w5163 -> [w5168 w5201]
              tunnel: w5162 -> [w5167 w5200]
              tunnel: w5161 -> [w5166 w5199]
              tunnel: w5160 -> [w5165 _]
              tunnel: w5149 -> [_ w5198]
              tunnel: w5159 -> [_ w5197]
              tunnel: w5158 -> [_ w5196]
              tunnel: w5157 -> [_ w5195]
              tunnel: w5156 -> [_ w5194]
              tunnel: w5155 -> [_ w5193]
              tunnel: w5154 -> [_ w5192]
              tunnel: w5153 -> [_ w5191]
              tunnel: w5152 -> [_ w5190]
              tunnel: w5151 -> [_ w5189]
              tunnel: w5150 -> [_ w5188]
              tunnel: "TO (string):" -> [w5164 _]
              frame #0 {
                # "mail test"
                n2819 = case shown="True" w5165 {
                  tunnel: w5168 -> [_ w5172]
                  tunnel: w5164 -> [_ w5171]
                  tunnel: w5167 -> [_ w5170]
                  tunnel: w5166 -> [_ w5169]
                  frame False {
                  }
                  frame True {
                    n2820 = stacked-sequence {
                      seq-local: [_ _ w5182 _] -> [_ _ _ w5183]
                      tunnel: w5172 -> [w5175 _ _ w5187]
                      tunnel: w5171 -> [_ _ w5180 _]
                      tunnel: w5170 -> [_ _ w5178 _]
                      tunnel: w5169 -> [_ _ w5179 _]
                      frame #0 {
                        n2821 = Bundle(cluster=w5175, "TEST MAIL STATUS"="TEST START") -> (w5173:T7)  [unwired: 6 in]
                        n2822 = local write "MAIL SETTINGS"(w5173) -> ()
                      }
                      frame #1 {
                        n2823 = Wait (ms)(milliseconds to wait=500) -> ()  [unwired: 1 out]
                      }
                      frame #2 {
                        n2824 = call "sub vi - send mail v5.vi"("TO:"=w5180, "subject"="MAIL TEST FROM LAB PANEL", "from"=w5179, "out going server"=w5178, "message"="TEST MESSAGE") -> ("error out"=w5182:errorcluster)  [unwired: 10 in]
                      }
                      frame #3 {
                        n2825 = Bundle(cluster=w5187, "TEST MAIL"=FALSE, "TEST MAIL STATUS"="TEST END", "mail error"=w5183) -> (w5185:T7)  [unwired: 4 in]
                        n2826 = local write "MAIL SETTINGS"(w5185) -> ()
                      }
                    }
                  }
                }
              }
              frame #1 {
                # "mail report"
                n2827 = stacked-sequence {
                  seq-local: [_ w5245 _ _] -> [_ _ _ w5435]
                  seq-local: [_ _ w5348 _] -> [_ _ _ w5425]
                  seq-local: [w5212 _ _ _] -> [_ w5262 _ _]
                  seq-local: [w5211 _ _ _] -> [_ w5261 _ _]
                  seq-local: [w5209 _ _ _] -> [_ w5259 _ _]
                  seq-local: [w5210 _ _ _] -> [_ w5260 _ _]
                  seq-local: [w5208 _ _ _] -> [_ w5258 _ _]
                  seq-local: [w5207 _ _ _] -> [_ w5253 _ _]
                  seq-local: [w5206 _ _ _] -> [_ w5254 _ _]
                  seq-local: [w5205 _ _ _] -> [_ w5255 _ _]
                  seq-local: [w5204 _ _ _] -> [_ w5256 _ _]
                  seq-local: [w5203 _ _ _] -> [_ w5257 _ _]
                  tunnel: w5202 -> [_ _ _ w5436]
                  tunnel: w5201 -> [_ _ _ w5419]
                  tunnel: w5200 -> [_ _ _ w5433]
                  tunnel: w5199 -> [_ _ _ w5432]
                  tunnel: w5198 -> [w5243 _ _ w5427]
                  tunnel: w5197 -> [_ _ w5378 _]
                  tunnel: w5196 -> [_ _ w5375 _]
                  tunnel: w5195 -> [_ _ w5374 _]
                  tunnel: w5194 -> [_ _ w5373 _]
                  tunnel: w5193 -> [_ _ w5372 _]
                  tunnel: w5192 -> [_ _ w5371 _]
                  tunnel: w5191 -> [_ _ w5370 _]
                  tunnel: w5190 -> [_ _ w5369 _]
                  tunnel: w5189 -> [_ _ w5368 _]
                  tunnel: w5188 -> [_ _ w5367 _]
                  frame #0 {
                    n2828 = case shown="False" w5243 {
                      frame False {
                        n2829 = local write "mail control"("") -> ()
                      }
                      frame True {
                      }
                    }
                    n2830 = local read "SET LAB01-1"() -> (w5242:T5)
                    n2831 = local read "SET LAB01-2"() -> (w5241:T5)
                    n2832 = local read "SET LAB02-1"() -> (w5240:T5)
                    n2833 = local read "SET LAB02-2"() -> (w5239:T5)
                    n2834 = local read "SET LAB03-1"() -> (w5238:T5)
                    n2835 = local read "SET LAB04-1"() -> (w5236:T5)
                    n2836 = local read "SET LAB05-1"() -> (w5234:T5)
                    n2837 = local read "SET LAB03-2"() -> (w5237:T5)
                    n2838 = local read "SET LAB04-2"() -> (w5235:T5)
                    n2839 = local read "SET LAB05-2"() -> (w5233:T5)
                    n2840 = Unbundle(w5238) -> ("DESCRIPTION"=w5218:string)  [unwired: 4 out]
                    n2841 = Unbundle(w5237) -> ("DESCRIPTION"=w5217:string)  [unwired: 4 out]
                    n2842 = Unbundle(w5236) -> ("DESCRIPTION"=w5216:string)  [unwired: 4 out]
                    n2843 = Unbundle(w5233) -> ("DESCRIPTION"=w5213:string)  [unwired: 4 out]
                    n2844 = Unbundle(w5239) -> ("DESCRIPTION"=w5219:string)  [unwired: 4 out]
                    n2845 = Unbundle(w5235) -> ("DESCRIPTION"=w5215:string)  [unwired: 4 out]
                    n2846 = Unbundle(w5242) -> ("DESCRIPTION"=w5231:string)  [unwired: 4 out]
                    n2847 = Unbundle(w5240) -> ("DESCRIPTION"=w5220:string)  [unwired: 4 out]
                    n2848 = Unbundle(w5234) -> ("DESCRIPTION"=w5214:string)  [unwired: 4 out]
                    n2849 = Unbundle(w5241) -> ("DESCRIPTION"=w5221:string)  [unwired: 4 out]
                    n2850 = Concatenate Strings("[LAB05-2/", w5213) -> (w5203:string)
                    n2851 = Concatenate Strings("[LAB05-1/", w5214) -> (w5204:string)
                    n2852 = Concatenate Strings("[LAB04-2/", w5215) -> (w5205:string)
                    n2853 = Concatenate Strings("[LAB03-2/", w5217) -> (w5207:string)
                    n2854 = Concatenate Strings("[LAB04-1/", w5216) -> (w5206:string)
                    n2855 = Concatenate Strings("[LAB03-1/", w5218) -> (w5208:string)
                    n2856 = Concatenate Strings("[LAB01-2/", w5221) -> (w5211:string)
                    n2857 = Concatenate Strings("[LAB02-2/", w5219) -> (w5209:string)
                    n2858 = Concatenate Strings("[LAB01-1/", w5231) -> (w5212:string)
                    n2859 = Concatenate Strings("[LAB02-1/", w5220) -> (w5210:string)
                  }
                  frame #1 {
                    w5266 = "/"
                    w5267 = 2.0
                    n2860 = local read "DISP LAB01-2"() -> (w5346:T4)
                    n2861 = local read "DISP LAB01-1"() -> (w5347:T4)
                    n2862 = local read "DISP LAB02-1"() -> (w5345:T4)
                    n2863 = local read "DISP LAB03-2"() -> (w5342:T4)
                    n2864 = local read "DISP LAB02-2"() -> (w5344:T4)
                    n2865 = local read "DISP LAB03-1"() -> (w5343:T4)
                    n2866 = local read "DISP LAB04-2"() -> (w5340:T4)
                    n2867 = local read "DISP LAB04-1"() -> (w5341:T4)
                    n2868 = local read "DISP LAB05-1"() -> (w5339:T4)
                    n2869 = local read "DISP LAB05-2"() -> (w5338:T4)
                    n2870 = Unbundle(w5346) -> ("CYCLE"=w5330:dbl, "MINS"=w5329:dbl, "STATUS"=w5326:string)
                    n2871 = Unbundle(w5347) -> ("CYCLE"=w5335:dbl, "MINS"=w5334:dbl, "STATUS"=w5331:string)
                    n2872 = Unbundle(w5345) -> ("CYCLE"=w5323:dbl, "MINS"=w5322:dbl, "STATUS"=w5321:string)
                    n2873 = Unbundle(w5342) -> ("CYCLE"=w5310:dbl, "MINS"=w5309:dbl, "STATUS"=w5306:string)
                    n2874 = Unbundle(w5343) -> ("CYCLE"=w5315:dbl, "MINS"=w5314:dbl, "STATUS"=w5311:string)
                    n2875 = Unbundle(w5344) -> ("CYCLE"=w5320:dbl, "MINS"=w5319:dbl, "STATUS"=w5316:string)
                    n2876 = Unbundle(w5341) -> ("CYCLE"=w5305:dbl, "MINS"=w5304:dbl, "STATUS"=w5301:string)
                    n2877 = Unbundle(w5340) -> ("CYCLE"=w5300:dbl, "MINS"=w5299:dbl, "STATUS"=w5296:string)
                    n2878 = Unbundle(w5339) -> ("CYCLE"=w5295:dbl, "MINS"=w5294:dbl, "STATUS"=w5291:string)
                    n2879 = Unbundle(w5338) -> ("CYCLE"=w5337:dbl, "MINS"=w5336:dbl, "STATUS"=w5288:string)
